vi "dataset.update_commit.vi"(8 "error in":errorcluster, 11 "DatasetUpdateStaging in":refnum<class "DatasetUpdateStaging.lvclass">) -> (0 "error out":errorcluster, 3 "DatasetUpdateStaging out":refnum<class "DatasetUpdateStaging.lvclass">)   [LabVIEW 2020, in "DatasetUpdateStaging.lvclass"]
doc: "Applies the staged update to the dataset with the given RID and returns a handle to the updated dataset."
uses:
  DatasetUpdateStaging.lvclass
  DatasetUpdateStaging.lvclass/DatasetUpdateStaging.ctl
  client.lvlib
panel:
  out "out_dataset out":i32
  in  "rid":string
  in  "staging":i32
  in  "out_dataset":i32
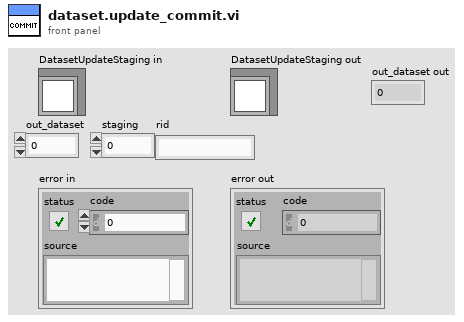
[diagram p1: front panel]
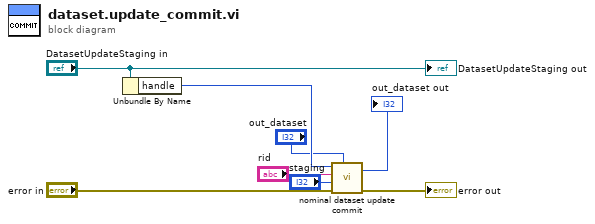
[diagram p0: block diagram]
diagram:
  n1 = Unbundle By Name("DatasetUpdateStaging in") -> ("handle"=w6:i32)
  n2 = call "nominal dataset update commit.vi"("out_dataset"="out_dataset", "error in (no error)"="error in", "staging"="staging", "rid"="rid", "client"=w6) -> ("error out"=→"error out":errorcluster, "out_dataset out"=→"out_dataset out":i32)  [unwired: 4 in, 1 out]
  "DatasetUpdateStaging out" <- "DatasetUpdateStaging in"
